vi "Tx RT Hardware Info.vi"(8 "error in":errorcluster, 10 "Reply Payload":T1={"Module ID"=-1, "Hardware Information"=variant(cluster{"Serial Hardware Info JSON Format":cluster{"Command":string, "SubCmd":string, "Channel":string[]}, "Hardware Info JSON Format":cluster{"Command":string, "SubCmd":string, "Input":string[], "Output":string[]}, "Hardware Info JSON Format":cluster{"Command":string, "SubCmd":string, "Input":string[], "Output":string[]}, "Ethernet IP Address JSON Format":cluster{"Command":string, "SubCmd":string, "IP":string[]}} {"Serial Hardware Info JSON Format"={"Command"="", "SubCmd"="", "Channel"=[]}, "Hardware Info JSON Format"={"Command"="", "SubCmd"="", "Input"=[], "Output"=[]}, "Hardware Info JSON Format"={"Command"="", "SubCmd"="", "Input"=[], "Output"=[]}, "Ethernet IP Address JSON Format"={"Command"="", "SubCmd"="", "IP"=[]}}), "error"={"status"=FALSE, "code"=0, "source"=""}}) -> (0 "error out":errorcluster)   [LabVIEW 2021, in "RT Acquisition Engine.lvlib"]
doc: "This Round trip event will request the hardware information from the Realtime and once the response has been received from the Realtime that response has been broadcasted to all the module's who register's this module reference.\n_____\nCreated using DQMH Event Scripter 7.0.1.1316."
uses:
  RT Acquisition Engine.lvlib
  Hardware Info (Reply Payload)--cluster.ctl
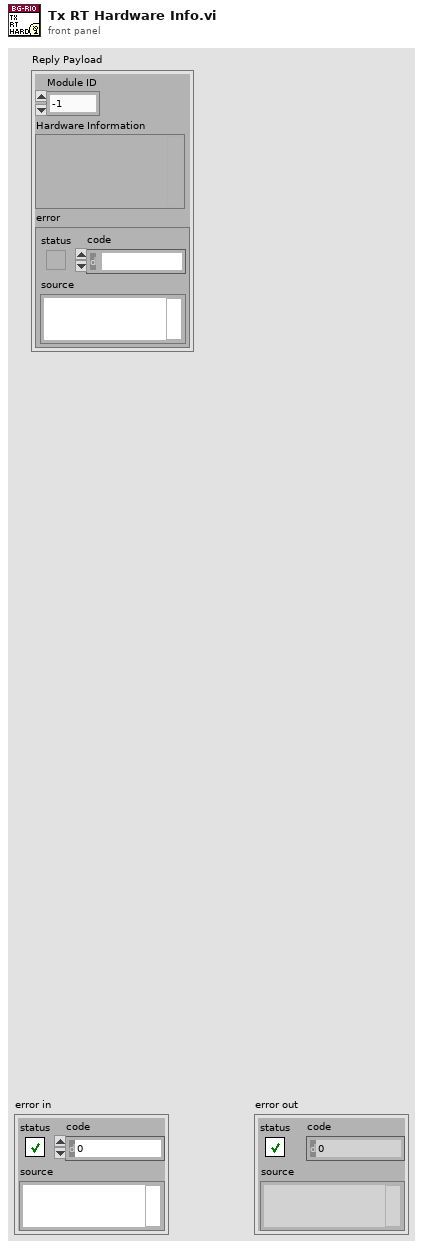
[diagram p1: front panel]
types:
  T1 = typedef "RT Acquisition Engine.lvlib/Hardware Info (Reply Payload)--cluster.ctl" = cluster{"Module ID":i32, "Hardware Information":variant, "error":errorcluster}
  T2 = typedef "RT Acquisition Engine.lvlib/Broadcast Events--cluster.ctl" = cluster{"Module Did Init":refnum<user-event>, "Status Updated":refnum<user-event>, "Error Reported":refnum<user-event>, "Module Did Stop":refnum<user-event>, "Update Module Execution Status":refnum<user-event>, "RT Connection Status":refnum<user-event>, "Tx RT Hardware Info":refnum<user-event>, "DO Data's":refnum<user-event>, "AI-Info":refnum<user-event>}
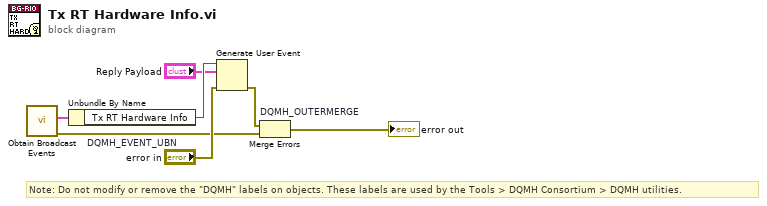
[diagram p0: block diagram]
diagram:
  # "Note: Do not modify or remove the \"DQMH\" labels on objects. These labels are used by the Tools > DQMH Consortium > DQMH utilities."
  n1 = call "Obtain Broadcast Events.vi"() -> ("error out"=w3:errorcluster, "RT Acquisition Engine Broadcast Events"=w2:T2)  [unwired: 10 in]
  n2 = Unbundle By Name "DQMH_EVENT_UBN"(w2) -> ("Tx RT Hardware Info"=w5:refnum<user-event>)
  n3 = Generate User Event(user event=w5, event data cluster="Reply Payload", error in="error in") -> (error out=w4:errorcluster)  [unwired: 1 in, 1 out]
  n4 = Merge Errors "DQMH_OUTERMERGE"(w4, w3) -> (→"error out":errorcluster)
